vi "Get Position.vi"(10 "Side":enum16{"Left", "Right"}(ring), 11 "drive in":refnum<class "drive.lvclass">) -> (1 "Side":enum16{"Left", "Right"}(ring), 2 "Position":dbl, 3 "drive out":refnum<class "drive.lvclass">)   [LabVIEW 2015, in "drive.lvclass"]
uses:
  drive.lvclass
  drive.lvclass/drive.ctl
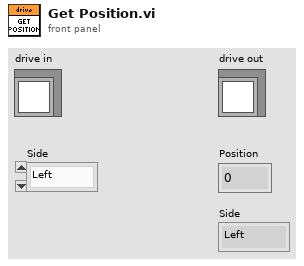
[diagram p1: front panel]
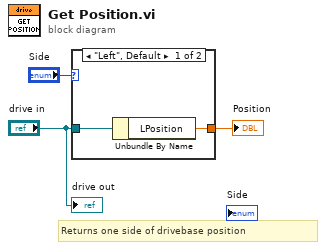
[diagram p0: block diagram]
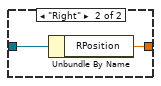
[diagram p2: hidden frame]
diagram:
  # "Returns one side of drivebase position"
  n1 = case shown="\"Left\", Default" "Side" {
    tunnel: "drive in" -> [w5 w6]
    tunnel: [w4 w7] -> w2
    frame "Left", Default {
      n2 = Unbundle By Name(w5) -> ("LPosition"=w4:dbl)
    }
    frame "Right" {
      n3 = Unbundle By Name(w6) -> ("RPosition"=w7:dbl)
    }
  }
  "Position" <- w2
  "drive out" <- "drive in"
